vi "Write I2C.vi"(8 "error in (no error)":errorcluster, 10 "LINX I2C":refnum<class "LINX I2C.lvclass">, 11 "LINX-ADS1015 in":refnum<class "LINX-ADS1X15.lvclass">) -> (0 "error out":errorcluster, 3 "LINX-ADS1015 out":refnum<class "LINX-ADS1X15.lvclass">)   [LabVIEW 2020, in "LINX-ADS1X15.lvclass"]
uses:
  LINX-ADS1X15.lvclass
  LINX I2C/LINX I2C.lvclass
  LINX-ADS1X15.lvclass/LINX-ADS1X15.ctl
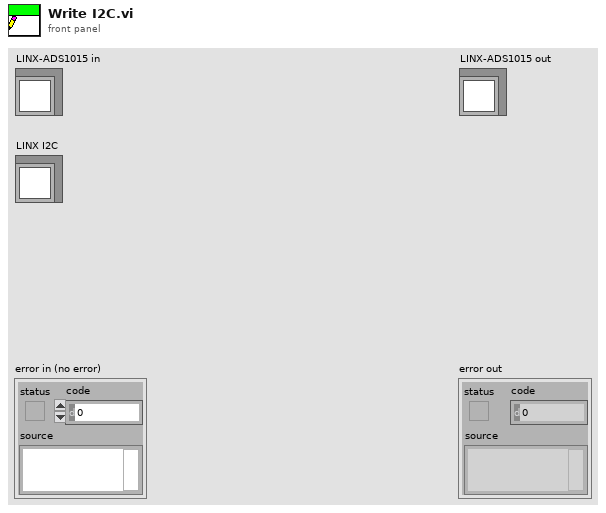
[diagram p1: front panel]
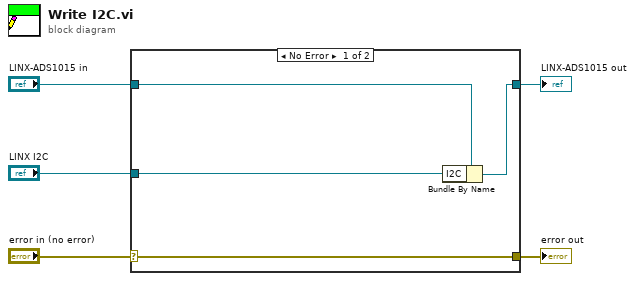
[diagram p0: block diagram]
diagram:
  n1 = case shown="No Error" "error in (no error)" {
    selector: "error in (no error)" -> [w9 w10]
    tunnel: [w9 w10] -> w4
    tunnel: [w7 w11] -> w2
    tunnel: "LINX-ADS1015 in" -> [w8 w11]
    tunnel: "LINX I2C" -> [w6 _]
    frame No Error {
      n2 = Bundle By Name(cluster=w8, "I2C"=w6) -> (w7:refnum<class "LINX-ADS1X15.lvclass">)
    }
    frame Error {
    }
  }
  "error out" <- w4
  "LINX-ADS1015 out" <- w2
